vi "Get NOK Counter.vi"(8 "error in (no error)":errorcluster) -> (0 "error out":errorcluster, 3 "NOK_Counter":u32)   [LabVIEW 2023, in "Counters.lvlib"]
uses:
  Counters.lvlib
  <vilib>/Utility/config.llb/Read Key (U32).vi
  <vilib>/Utility/config.llb/NI_LVConfig.lvlib
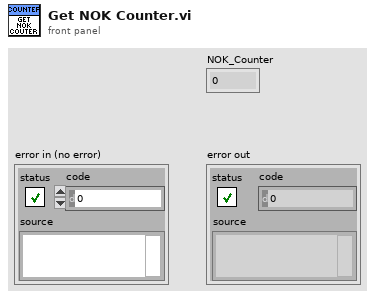
[diagram p1: front panel]
types:
  T1 = typedef "NI_LVConfig.lvlib/Config Data RefNum.ctl" = refnum<k1>
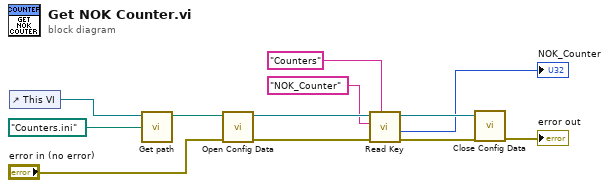
[diagram p0: block diagram]
diagram:
  n1 = control-ref of="This VI"() -> (w1:refnum<vi>)
  n2 = call "Get path.vi"("File mame"=path "Counters.ini" ("configuration file path"), "VI in"=w1) -> ("File path"=w3:path)  [unwired: 9 in]
  n3 = call <vilib>:"Open Config Data.vi"("error in (no error)"="error in (no error)", "configuration file path"=w3) -> ("error out"=w9:errorcluster, "refnum"=w10:T1)  [unwired: 7 in, 1 out]
  n4 = call-poly <vilib>:"Read Key.vi"("section"="Counters", "error in (no error)"=w9, "key"="NOK_Counter", "refnum"=w10) -> ("error out"=w7:errorcluster, "value"=→"NOK_Counter":u32, "refnum out"=w8:T1)  [unwired: 4 in, 1 out]
  n5 = call <vilib>:"Close Config Data.vi"("error in (no error)"=w7, "refnum"=w8) -> ("error out"=→"error out":errorcluster)  [unwired: 8 in, 1 out]
